vi "BToUInt.vi"(1 "Binary Array":i32[](array[numeric])) -> (0 "Unsigned  Integer":i32)   [LabVIEW 2018]
doc: "Converts Binary Stream (first element LSB) to Unisgned Int"
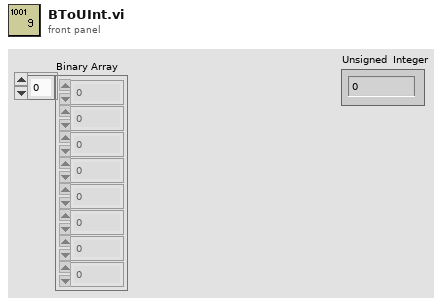
[diagram p1: front panel]
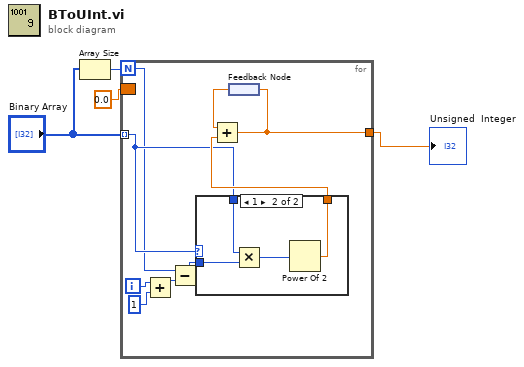
[diagram p0: block diagram]
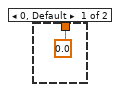
[diagram p2: hidden frame]
diagram:
  n1 = Array Size(array="Binary Array") -> (size(s)=w4:i32)
  n2 = for {
    N: w4 -> [w9]
    tunnel: "Binary Array" -> [w10] mode=indexing
    tunnel: [w12] -> w2
    border: 0.0 -> [_]
    i -> [w6]
    n3 = Add(x=w6, y=1) -> (x+y=w7:i32)
    n4 = Subtract(x=w9, y=w7) -> (x-y=w8:i32)
    n5 = case shown="1" w10 {
      tunnel: w8 -> [_ w18]
      tunnel: w10 -> [_ w17]
      tunnel: [0.0 w15] -> w11
      frame 0, Default {
      }
      frame 1 {
        n6 = Multiply(x=w17, y=w18) -> (x*y=w16:i32)
        n7 = Power Of 2(x=w16) -> (2^x=w15:dbl)
      }
    }
    n8 = feedback #1() -> (w13:dbl)
    n9 = Add(x=w13, y=w11) -> (x+y=w12:dbl)
    n10 = feedback-in #1(w12) -> ()
  }
  "Unsigned  Integer" <- w2
